vi "Test Serial Session.vi"() -> ()   [LabVIEW 2014]
uses:
  Reusable/Session Log/System Log.lvclass
  Reusable/Session APIs/File Access/Config Data/Config Data.lvclass
  Session/FPGA Serial Session.lvclass
  Devices/PPT/PPT.lvclass
  Session/Raw FPGA/FPGA Session.lvclass
  Devices/Vaisala Probe/Vaisala.lvclass
  Reusable/Session Log/System Log.lvclass/System Log.ctl
  Reusable/Session APIs/File Access/Config Data/Config Data.lvclass/Config Data.ctl
  Devices/Vaisala Probe/Vaisala.lvclass/Vaisala.ctl
  <vilib>/Platform/TimedLoop/XDataNode/timing_clust.ctl
  <vilib>/Platform/TimedLoop/XDataNode/nitl_modes.ctl
  <vilib>/Platform/TimedLoop/XDataNode/wakeup.ctl
  Session/FPGA Serial Session.lvclass/FPGA Serial Session.ctl
  Reusable/Session APIs/Text Communication/Text Device Session.lvclass/Text Device Session.ctl
  Devices/Configurable Device/Configurable Device.lvclass/Configurable Device.ctl
  Reusable/Data/Array Data/Single 1-D/Single_Array.lvclass
  Session/Write fpgaSession.vi
  Reusable/Session APIs/Text Communication/Write hSysLog.vi
  Devices/Configurable Device/Write Handle.vi
  Reusable/Session Log/Accessors/Write Main Path.vi
  Reusable/Session APIs/File Access/Config Data/Accessors/Write Cfg Path.vi
  Devices/Vaisala Probe/Accessors/Write ID.vi
  Devices/Vaisala Probe/Accessors/Write hSession.vi
  <vilib>/Platform/TimedLoop/XDataNode/XDataNode.xnode
  <userlib>/_Session Fwk/Session - Root.lvclass
  <vilib>/Platform/TimedLoop/XDataNode/XDNodeRunTimeDep.lvlib
panel:
  out "Array 2":errorcluster[](array[cluster])
  out "Array":errorcluster[](array[cluster])
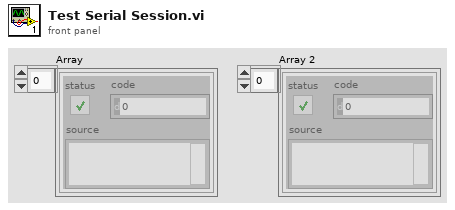
[diagram p1: front panel]
types:
  T1 = typedef "Session - Root.lvclass/Session Handle.ctl" = refnum<data-value>
  T2 = typedef "XDNodeRunTimeDep.lvlib/timing_clust.ctl" = cluster{"Expected End [f-1]":u64, "Actual End [f-1]":u64, "Finished Late? [f-1]":bool, "Expected End [i-1]":u64, "Actual End [i-1]":u64, "Finished Late? [i-1]":bool, "Expected Start [i]":u64, "Actual Start [i]":u64, "Expected Start [f]":u64, "Actual Start [f]":u64, "Source Name":string, "Structure Name":string, "Period":i64, "Deadline":i64, "Offset":i64, "Start":i64, "Priority":i32, "Timeout":i32, "Mode":T3, "Wakeup Reason":T4, "Error":errorcluster, "Source Type":string, "Secondary Source Type":string, "Global End Time":u64, "Global Start Time":u64, "Frame Duration":u64, "Iteration Duration":u64, "Assigned CPU":i32, "I/O Scan Engine Mode":u32}
  T3 = typedef "XDNodeRunTimeDep.lvlib/nitl_modes.ctl" = enum32{"No Change", "Process missed periods, maintain original phase", "Discard missed periods, maintain original phase", "Process missed periods, ignore original phase", "Discard missed periods, ignore original phase"}
  T4 = typedef "XDNodeRunTimeDep.lvlib/wakeup.ctl" = enum32{"Normal", "Aborted", "Asynchronous wakeup", "Timing source error", "Timed loop error", "Timeout"}
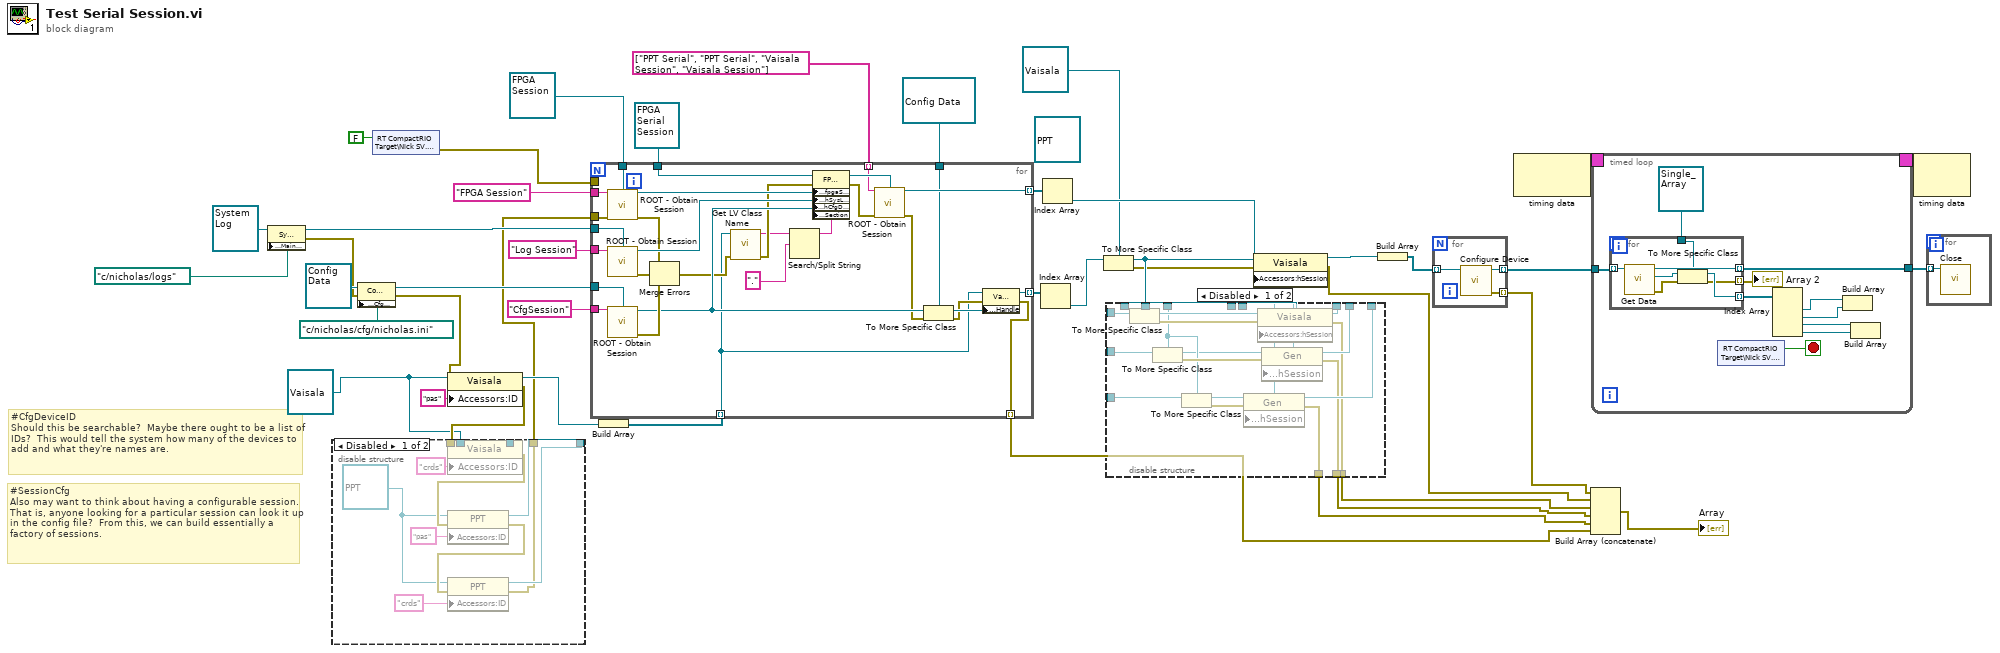
[diagram p0: block diagram]
diagram:
  w2 = refnum<class "Vaisala.lvclass"> refnum ("Vaisala")
  (unwired) refnum<class "PPT.lvclass"> refnum ("PPT")
  # "#SessionCfg\nAlso may want to think about having a configurable session.  That is, anyone looking for a particular session can look it up in the config file?  From this, we can build essentially a factory of sessions."
  # "#CfgDeviceID\nShould this be searchable?  Maybe there ought to be a list of IDs?  This would tell the system how many of the devices to add and what they're names are."
  n1 = property class="Sys Log"(reference=refnum<class "System Log.lvclass"> refnum ("Sys Log"), "Accessors:Main Path"=path "c:/nicholas/logs" ("Main Path")) -> (reference out=w18:refnum<class "System Log.lvclass">, error out=w14:errorcluster)  [unwired: 1 in]
  n2 = property class="Config Data"(reference=refnum<class "Config Data.lvclass"> refnum ("Config Data"), error in=w14, "Accessors:Cfg Path"=path "c:/nicholas/cfg/nicholas.ini" ("Cfg Path")) -> (reference out=w20:refnum<class "Config Data.lvclass">, error out=w13:errorcluster)
  n3 = shared-variable "RT CompactRIO Target\\Nick SV.lvlib\\Stop"(FALSE ("Stop")) -> (error out=w15:errorcluster)  [unwired: 1 in]
  n4 = property class="Vaisala"(reference=w2, error in=w13, "Accessors:ID"="pas" ("ID")) -> (reference out=w34:refnum<class "Vaisala.lvclass">, error out=w12:errorcluster)
  n5 = disable-structure shown="Disabled" {
    disable-tunnel: w2 -> [w55 _]
    disable-tunnel: [w51 _] -> _
    disable-tunnel: [w50 _] -> _
    disable-tunnel: [w49 _] -> _
    disable-tunnel: w12 -> [w48 _]
    disable-tunnel: [w45 _] -> w11
    frame Disabled {
      w44 = refnum<class "PPT.lvclass"> refnum ("PPT")
      n6 = property class="Vaisala"(reference=w55, error in=w48, "Accessors:ID"="crds" ("ID")) -> (reference out=w51:refnum<class "Vaisala.lvclass">, error out=w47:errorcluster)
      n7 = property class="PPT"(reference=w44, error in=w47, "Accessors:ID"="pas" ("ID")) -> (reference out=w50:refnum<class "PPT.lvclass">, error out=w46:errorcluster)
      n8 = property class="PPT"(reference=w44, error in=w46, "Accessors:ID"="crds" ("ID")) -> (reference out=w49:refnum<class "PPT.lvclass">, error out=w45:errorcluster)
    }
    frame Enabled {
    }
  }
  n9 = Build Array(w34) -> (w36:refnum<class "Vaisala.lvclass">[])
  n10 = for {
    tunnel: w18 -> [w85]
    tunnel: "Log Session" ("Session Name ()") -> [w84]
    tunnel: "FPGA Session" ("Session Name ()") -> [w83]
    tunnel: w20 -> [w82]
    tunnel: "CfgSession" ("Session Name ()") -> [w81]
    tunnel: refnum<class "FPGA Serial Session.lvclass"> refnum ("FPGA Serial Session.lvclass") -> [w79]
    tunnel: w36 -> [w60] mode=indexing
    tunnel: [w70] -> w28 mode=indexing
    tunnel: [w69] -> w33 mode=indexing
    tunnel: refnum<data-value> refnum ("Session Handle") -> [w66]
    tunnel: [w58] -> w5 mode=indexing
    tunnel: string[] ["PPT Serial", "PPT Serial", "Vaisala Session", "Vaisala Session"] -> [w59] mode=indexing
    tunnel: w15 -> [_]
    tunnel: w11 -> [w57]
    tunnel: refnum<class "FPGA Session.lvclass"> refnum ("FPGA Session") -> [w56]
    n11 = call <userlib>:"ROOT - Obtain Session.vi"("Session Name ()"=w83, "OBJ - Session"=w56, "error in (no error)"=w57) -> ("Session Handle"=w80:T1, "error out"=w76:errorcluster)  [unwired: 10 in, 1 out]
    n12 = call <userlib>:"ROOT - Obtain Session.vi"("Session Name ()"=w84, "OBJ - Session"=w85) -> ("Session Handle"=w77:T1, "error out"=w75:errorcluster)  [unwired: 11 in, 1 out]
    n13 = call <userlib>:"ROOT - Obtain Session.vi"("Session Name ()"=w81, "OBJ - Session"=w82) -> ("Session Handle"=w72:T1, "error out"=w74:errorcluster)  [unwired: 11 in, 1 out]
    n14 = Merge Errors(w76, w75, w74) -> (w65:errorcluster)
    n15 = call <vilib>:"Get LV Class Name.vi"("error in (no error)"=w65, "object"=w60) -> ("error out"=w64:errorcluster, "class name"=w62:string)  [unwired: 8 in]
    n16 = Search/Split String(string=w62, search string/char (-)="." ("regular expression")) -> (substring before match=w61:string)  [unwired: 1 in, 2 out]
    n17 = property class="FPGA Serial Session"(reference=w79, error in=w64, "Accessors:fpgaSession"=w80, "Accessors:hSysLog"=w77, "Accessors:hCfgData"=w72, "Accessors:Section"=w61) -> (reference out=w78:refnum<class "FPGA Serial Session.lvclass">, error out=w73:errorcluster)
    n18 = call <userlib>:"ROOT - Obtain Session.vi"("Session Name ()"=w59, "OBJ - Session"=w78, "error in (no error)"=w73) -> ("Session Handle"=w70:T1, "error out"=w68:errorcluster)  [unwired: 10 in, 1 out]
    n19 = To More Specific Class(target class=w66, reference=w72, error in=w68) -> (specific class reference=w71:refnum<data-value>, error out=w67:errorcluster)
    n20 = property class="Vaisala"(reference=w60, error in=w67, "Accessors:Handle"=w71) -> (reference out=w69:refnum<class "Vaisala.lvclass">, error out=w58:errorcluster)
  }
  n21 = Index Array(array=w33) -> (element=w32:refnum<class "Vaisala.lvclass">)  [unwired: 1 in]
  n22 = Index Array(array=w28) -> (element=w27:T1)  [unwired: 1 in]
  n23 = To More Specific Class(target class=refnum<class "Vaisala.lvclass"> refnum ("Vaisala"), reference=w32) -> (specific class reference=w31:refnum<class "Vaisala.lvclass">, error out=w22:errorcluster)  [unwired: 1 in]
  n24 = disable-structure shown="Disabled" {
    disable-tunnel: _ -> [w105 _]
    disable-tunnel: _ -> [w104 _]
    disable-tunnel: _ -> [w103 _]
    disable-tunnel: w31 -> [w102 _]
    disable-tunnel: [w99 _] -> _
    disable-tunnel: _ -> [w98 _]
    disable-tunnel: _ -> [w94 _]
    disable-tunnel: [w92 _] -> _
    disable-tunnel: [w91 _] -> _
    disable-tunnel: [w90 _] -> w8
    disable-tunnel: [w89 _] -> w7
    disable-tunnel: [w88 _] -> w6
    disable-tunnel: _ -> [w87 _]
    disable-tunnel: _ -> [w86 _]
    frame Disabled {
      n25 = To More Specific Class(target class=w102, reference=w105) -> (specific class reference=w101:refnum<class "Vaisala.lvclass">, error out=w95:errorcluster)  [unwired: 1 in]
      n26 = To More Specific Class(target class=w94, reference=w104) -> (specific class reference=w93:refnum<vi>, error out=w96:errorcluster)  [unwired: 1 in]
      n27 = To More Specific Class(target class=w94, reference=w103) -> (specific class reference=w100:refnum<vi>, error out=w97:errorcluster)  [unwired: 1 in]
      n28 = property class="Gen"(reference=w100, error in=w97, "Accessors:hSession"=w87) -> (reference out=w91:refnum<vi>, error out=w88:errorcluster)
      n29 = property class="Vaisala"(reference=w101, error in=w95, "Accessors:hSession"=w98) -> (reference out=w99:refnum<class "Vaisala.lvclass">, error out=w90:errorcluster)
      n30 = property class="Gen"(reference=w93, error in=w96, "Accessors:hSession"=w86) -> (reference out=w92:refnum<vi>, error out=w89:errorcluster)
    }
    frame Enabled {
    }
  }
  n31 = property class="Vaisala"(reference=w31, error in=w22, "Accessors:hSession"=w27) -> (reference out=w30:refnum<class "Vaisala.lvclass">, error out=w9:errorcluster)
  n32 = Build Array(w30) -> (w29:refnum<class "Vaisala.lvclass">[])
  n33 = for {
    tunnel: w29 -> [w108] mode=indexing
    tunnel: [w107] -> w25 mode=indexing
    tunnel: [w106] -> w10 mode=indexing
    n34 = call-dynamic "Configure Device.vi"("Vaisala Probe in"=w108) -> ("error out"=w106:errorcluster, "Vaisala Probe out"=w107:refnum<class "Vaisala.lvclass">)  [unwired: 9 in]
  }
  n35 = node-c288() -> (w43:T2)  [unwired: 1 in]
  n36 = Build Array (concatenate)(w10, w9, w8, w7, w6, w5) -> (→"Array":errorcluster[])
  n37 = timed-loop {
    tunnel: w25 -> [w118]
    tunnel: [w117] -> w24
    timing: w43 -> [_]
    timing-out: [_] -> w42
    stop <- w116 stop-if-true
    n38 = for {
      tunnel: w118 -> [w125] mode=indexing
      tunnel: [w124] -> w117 mode=indexing
      tunnel: refnum<class "Single_Array.lvclass"> refnum ("Base Data Lib:[SGL]") -> [w122]
      tunnel: [w121] -> w114 mode=indexing
      tunnel: [w119] -> w109 mode=indexing
      n39 = call-dynamic "Get Data.vi"("Cfg Dev in"=w125) -> ("error out"=w120:errorcluster, "Data"=w123:refnum<class "Data.lvclass">, "Cfg Dev out"=w124:refnum<class "Vaisala.lvclass">)  [unwired: 8 in]
      n40 = To More Specific Class(target class=w122, reference=w123, error in=w120) -> (specific class reference=w121:refnum<class "Single_Array.lvclass">, error out=w119:errorcluster)
    }
    "Array 2" <- w109
    n41 = shared-variable "RT CompactRIO Target\\Nick SV.lvlib\\Stop"() -> (w116:bool)  [unwired: 1 in, 1 out]
    n42 = Index Array(array=w114) -> (element #1=w113:refnum<class "Single_Array.lvclass">, element #2=w112:refnum<class "Single_Array.lvclass">, element #3=w111:refnum<class "Single_Array.lvclass">, element #4=w110:refnum<class "Single_Array.lvclass">)  [unwired: 4 in]
    n43 = Build Array(w113, w112) -> ()  [unwired: 1 out]
    n44 = Build Array(w111, w110) -> ()  [unwired: 1 out]
  }
  n45 = node-c288(w42) -> ()  [unwired: 1 out]
  n46 = for {
    tunnel: w24 -> [w128] mode=indexing
    n47 = call-dynamic "Close.vi"("Cfg Dev in"=w128) -> ()  [unwired: 9 in, 2 out]
  }
